vi "ChangeLevel (SubVI).vi"(10 "Array in":dbl[][](array[numeric]), 11 "Digital in":refnum<vi>) -> (3 "Array out":dbl[][](array[numeric]))   [LabVIEW 2014]
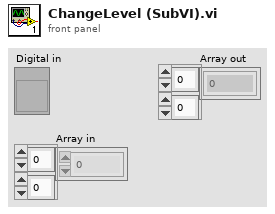
[diagram p1: front panel]
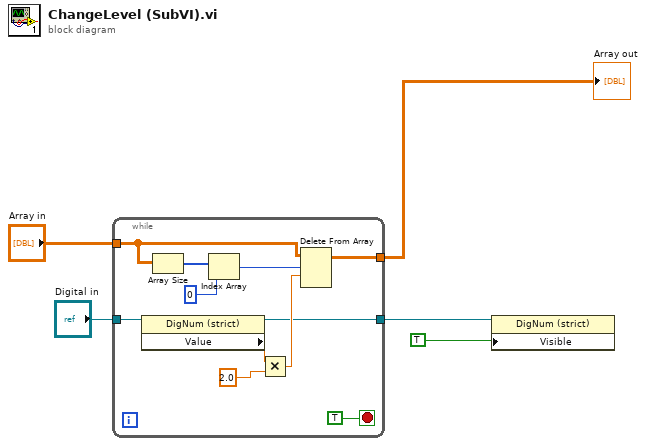
[diagram p0: block diagram]
diagram:
  n1 = while {
    tunnel: "Array in" -> [w11]
    tunnel: [w10] -> w5
    tunnel: "Digital in" -> [w7]
    tunnel: [w6] -> w2
    stop <- TRUE stop-if-true
    n2 = property class="DigNum (strict)"(reference=w7) -> (reference out=w6:refnum<vi>, "Value"=w9:dbl)  [unwired: 1 in, 1 out]
    n3 = Array Size(array=w11) -> (size(s)=w13:i32[])
    n4 = Index Array(array=w13, index=0) -> (element=w12:i32)
    n5 = Multiply(x=w9, y=2.0) -> (x*y=w14:dbl)
    n6 = Delete From Array(array=w11, length=w12, index (row)=w14) -> (array with subset deleted=w10:dbl[][])  [unwired: 1 in, 1 out]
  }
  "Array out" <- w5
  n7 = property class="DigNum (strict)"(reference=w2, "Visible"=TRUE) -> ()  [unwired: 1 in, 2 out]
